vi "LVClass_WavefrontCorrectorSet get general specification.vi"(0 "WavefrontCorrectorSet in":refnum<class "WavefrontCorrectorSet.lvclass">, 11 "error in (no error)":errorcluster) -> (4 "WavefrontCorrectorSet out":refnum<class "WavefrontCorrectorSet.lvclass">, 6 "ConfigMiroir":T1={"Mirror name"="", "Plugin name"="", "Serial number"="", "Revision"="", "Number of commands"=0, "Sleep after command apply (ms)"=0, "Has internal memory ?"=TRUE}, 15 "error out":errorcluster)   [LabVIEW 2020, in "WavefrontCorrectorSet.lvclass"]
doc: "WavefrontCorrector specifications getters.\n\n--------------------------------------------------------------------------------\n\n<B>wavefrontcorrector_setIn </B> : WavefrontCorrectorSet object.\n<B>wavefrontcorrector_setOut </B> : WavefrontCorrectorSet object.\n<B>driver_name </B> : Wavefront corrector driver name.\n<B>wavefrontcorrector_name </B> : Wavefront corrector pretty name.\n<B>wavefrontcorrector_serial_number</B> : Wavefront corrector serial number.\n<B>revision </B> : Wavefront corrector revision.\n<B>actuators_count </B> : Wavefront corrector actuators count.\n<B>min_sleep_after_movement </B> : Wavefront corrector actuators stabilization delay.\n<B>ErrorIn </B> : Error\n<B>ErrorOut </B> : Error\n\n--------------------------------------------------------------------------------"
uses:
  WavefrontCorrectorSet.lvclass
  WavefrontCorrectorSpecifications.ctl
  WavefrontCorrectorSet.lvclass/WavefrontCorrectorSet.ctl
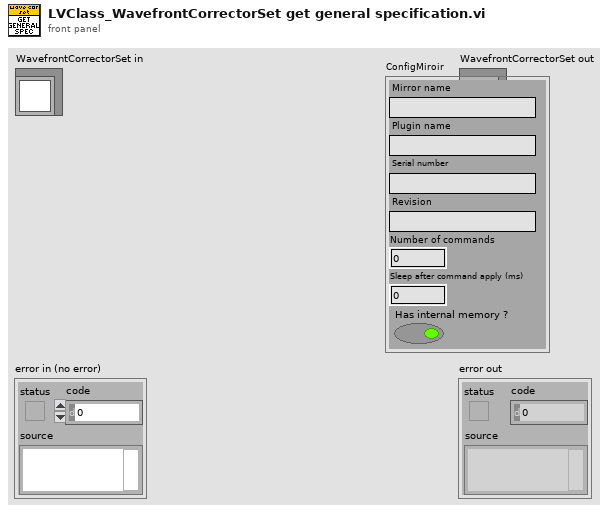
[diagram p1: front panel]
types:
  T1 = typedef "WavefrontCorrectorSpecifications.ctl" = cluster{"Mirror name":string, "Plugin name":string, "Serial number":string, "Revision":string, "Number of commands":i32, "Sleep after command apply (ms)":i32, "Has internal memory ?":bool}
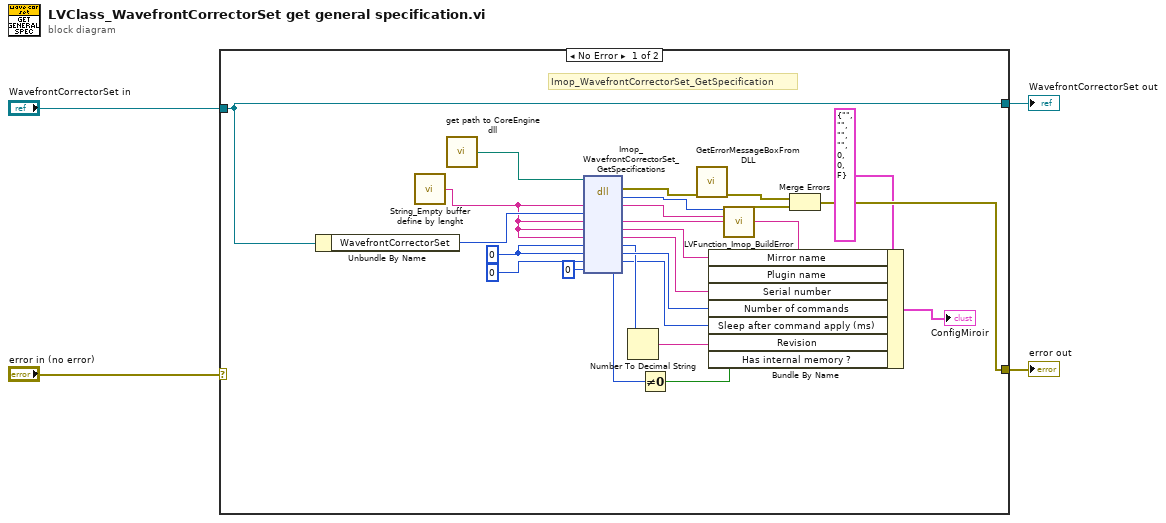
[diagram p0: block diagram]
diagram:
  n1 = case shown="No Error" "error in (no error)" {
    selector: "error in (no error)" -> [_ w30]
    tunnel: [w26 w30] -> w1
    tunnel: [w25 w29] -> w2
    tunnel: "WavefrontCorrectorSet in" -> [w25 w29]
    frame No Error {
      w11 = 0 ("nb_actuator")
      # "Imop_WavefrontCorrectorSet_GetSpecification"
      n2 = Unbundle By Name(w25) -> ("WavefrontCorrectorSet"=w23:i32)
      n3 = call "String_Empty buffer define by lenght.vi"() -> ("Empty buffer"=w19:string)  [unwired: 1 in]
      n4 = call "get path to CoreEngine dll.vi"() -> ("path to c_interface_vc100.dll"=w24:path)  [unwired: 12 in, 3 out]
      n5 = dll-call lib="D:/soft/HASO_v3/SVN_trunk/ImOpCoreEngine4_LV2011/DLLs/c_interface_vc100.dll" fn="Imop_WavefrontCorrectorSet_GetSpecifications"(path in=w24, "message"=w19, "WavefrontCorrectionSet"=w23, "driver_name"=w19, "WaveFrontCorrector_name"=w19, "WaveFrontCorrector_serial_number"=w19, "revision"=w11, "nb_actuator"=w11, "min_sleep_after_movement"=0, "Has internal memory"=u8 0) -> (error out=w22:errorcluster, "return type"=w21:i32, "message"=w20:string, "driver_name"=w12:string, "WaveFrontCorrector_name"=w16:string, "WaveFrontCorrector_serial_number"=w14:string, "revision"=w10:i32, "nb_actuator"=w13:i32, "min_sleep_after_movement"=w8:i32, "Has internal memory"=w7:u8)  [unwired: 3 in, 1 out]
      n6 = Number To Decimal String(number=w10) -> (decimal integer string=w9:string)  [unwired: 1 in]
      n7 = Not Equal To 0?(x=w7) -> (x != 0?=w6:bool)
      n8 = call "GetErrorMessageBoxFromDLL.vi"("error IN"=w22) -> ("error OUT"=w28:errorcluster)  [unwired: 10 in]
      n9 = Bundle By Name(cluster=T1 {"Mirror name"="", "Plugin name"="", "Serial number"="", "Revision"="", "Number of commands"=0, "Sleep after command apply (ms)"=0, "Has internal memory ?"=FALSE} ("ConfigMiroir"), "Mirror name"=w16, "Plugin name"=w12, "Serial number"=w14, "Number of commands"=w13, "Sleep after command apply (ms)"=w8, "Revision"=w9, "Has internal memory ?"=w6) -> (→"ConfigMiroir":T1)
      n10 = call "LVFunction_Imop_BuildError.vi"("code"=w21, "String to Prepend to source (\"\")"=w20) -> ("error out"=w27:errorcluster)  [unwired: 13 in]
      n11 = Merge Errors(w28, w27) -> (w26:errorcluster)
    }
    frame Error {
    }
  }
  "error out" <- w1
  "WavefrontCorrectorSet out" <- w2
